vi "例4.10-3 累加（while循环）反馈节点1.vi"() -> ()   [LabVIEW 2017]
panel:
  out "和":i32
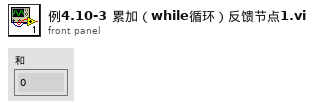
[diagram p1: front panel]
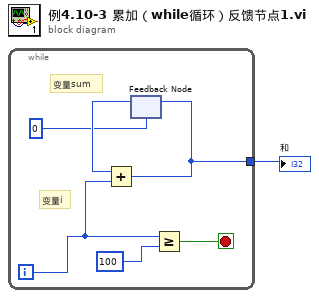
[diagram p0: block diagram]
diagram:
  n1 = while {
    tunnel: [w4] -> w1
    i -> [w5]
    stop <- w6 stop-if-true
    # "变量i"
    # "变量sum"
    n2 = feedback #1(0) -> (w3:i32)
    n3 = Add(x=w3, y=w5) -> (x+y=w4:i32)
    n4 = feedback-in #1(w4) -> ()
    n5 = Greater Or Equal?(x=w5, y=100) -> (x >= y?=w6:bool)
  }
  "和" <- w1
